vi "UpdateLowRateCount.vi"(7 "Qbus in":refnum<class "Qbus.lvclass">, 8 "error in (no error)":errorcluster, 10 "message value":variant, 11 "config":variant) -> (0 "error out":errorcluster, 3 "config out":variant)   [LabVIEW 2017, in "DataAccumulator.lvlib"]
uses:
  <vilib>/addons/InsightCM/Devices/Shared/Common/DataAccumulator/DataAccumulator.lvlib
  <vilib>/addons/Qbus/Qbus.lvclass
  <vilib>/addons/InsightCM/Devices/Shared/Common/DataAccumulator/controls/config.ctl
  <vilib>/addons/InsightCM/Devices/Shared/Common/DeviceHealth/controls/deviceHealthTag.ctl
  <vilib>/addons/InsightCM/Devices/Shared/Common/DeviceHealth/controls/SystemHealthTagEnum.ctl
  <vilib>/addons/InsightCM/MessageBus/Base/controls/Tag.ctl
  <vilib>/addons/InsightCM/MessageBus/Base/controls/KeyValuePair.ctl
  <vilib>/addons/InsightCM/MessageBus/Base/controls/TsTagValueString.ctl
  <vilib>/addons/InsightCM/MessageBus/Base/controls/TagValueUpdate.ctl
  <vilib>/addons/InsightCM/MessageBus/MessageLibrary/Tag/controls/TagUpdateTagValuesRoutedMessageBody.ctl
  <vilib>/addons/InsightCM/Devices/Shared/Common/ServerComm/ServerComm.lvlib
  <vilib>/addons/InsightCM/Devices/Shared/Common/DeviceHealth/DeviceHealth.lvlib
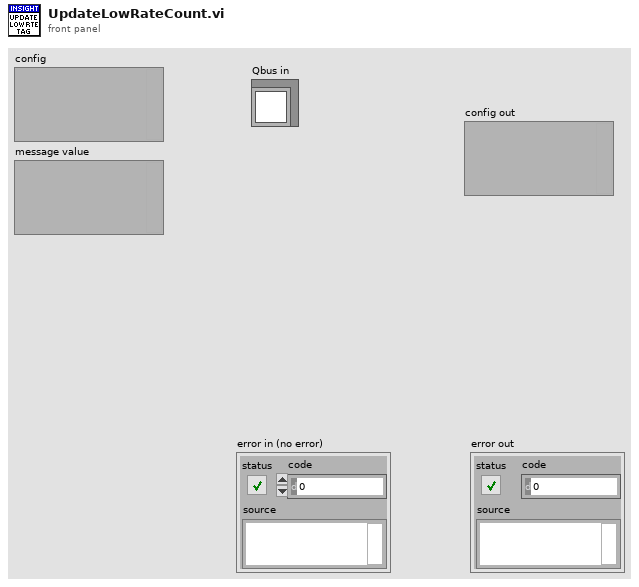
[diagram p1: front panel]
types:
  T1 = typedef "DataAccumulator.lvlib/config.ctl" = cluster{"Group":string, "BlockComplete":bool, "Ok To Start":bool, "Speed Ref Chan":string, "Current OpState":string, "MaxLowRateCPU(%)":dbl, "MaxLowRateMem(%)":dbl, "LowRateCount":i32, "LowRateCountTag":T2}
  T2 = typedef "DeviceHealth.lvlib/deviceHealthTag.ctl" = cluster{"SystemTags":T3, "TagId":string, "Tag":T4}
  T3 = typedef "DeviceHealth.lvlib/SystemHealthTagEnum.ctl" = enum16{"CPU Utilization", "Memory Utilization", "Disk Utilization", "Total Physical Memory", "Primary Disk Free", "Chassis Temperature", "LowRateCount"}
  T4 = typedef "Tag.ctl" = cluster{"Id":string, "Path":string, "Name":string, "Datatype":string, "Props":T5[], "Keywords":string[]}
  T5 = typedef "KeyValuePair.ctl" = cluster{"Key":string, "Value":string}
  T6 = typedef "TagValueUpdate.ctl" = cluster{"Tag":T4, "TsValue":T7}
  T7 = typedef "TsTagValueString.ctl" = cluster{"Value":string, "Timestamp":i64}
  T8 = typedef "TagUpdateTagValuesRoutedMessageBody.ctl" = cluster{"TagsValue":T6[]}
  T9 = typedef "Message.ctl" = cluster{"Header":T10, "Body":u8[]}
  T10 = typedef "MessageHeader.ctl" = cluster{"MessageName":string, "Timestamp":i64, "CorrelationId":string, "ContentType":string, "RoutingKey":string, "Properties":T5[]}
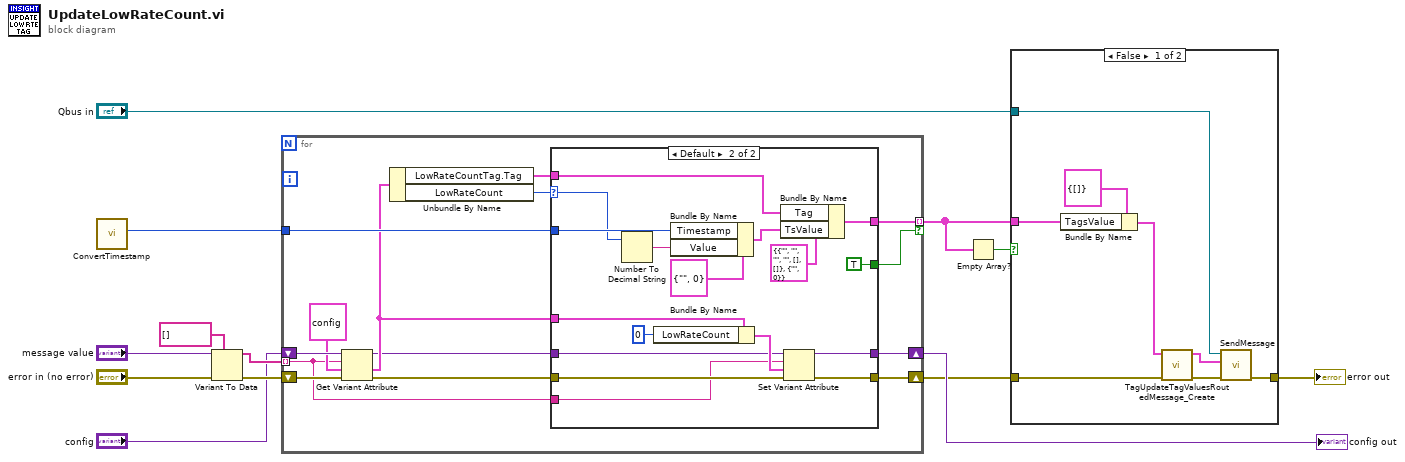
[diagram p0: block diagram]
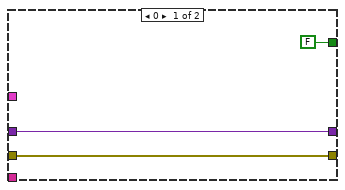
[diagram p2: hidden frame]
diagram:
  n1 = call <vilib>:"ConvertTimestamp.vi"() -> ("Timestamp out"=w3:i64)  [unwired: 11 in]
  n2 = Variant To Data(error in="error in (no error)", type=string[] [], Variant="message value") -> (data=w8:string[], error out=w10:errorcluster)
  n3 = for {
    shift-right: [w19] -> w2
    shift-left: w10 -> [w27]
    tunnel: w8 -> [w17] mode=indexing
    shift-right: [w18] -> w4
    shift-left: "config" -> [w26]
    tunnel: w3 -> [w24]
    tunnel: [w22] -> w1 mode=indexing if=w20
    n4 = Get Variant Attribute(Variant=w26, name=w17, default value (empty Variant)=T1 {"Group"="", "BlockComplete"=FALSE, "Ok To Start"=FALSE, "Speed Ref Chan"="", "Current OpState"="", "MaxLowRateCPU(%)"=0.0, "MaxLowRateMem(%)"=0.0, "LowRateCount"=0, "LowRateCountTag"={"SystemTags"=enum."CPU Utilization", "TagId"="", "Tag"={"Id"="", "Path"="", "Name"="", "Datatype"="", "Props"=[], "Keywords"=[]}}} ("Config"), error in=w27) -> (duplicate Variant=w15:variant, value=w16:T1, error out=w14:errorcluster)  [unwired: 1 out]
    n5 = Unbundle By Name(w16) -> ("LowRateCountTag.Tag"=w23:T4, "LowRateCount"=w21:i32)
    n6 = case shown="Default" w21 {
      selector: w21 -> [_ w39]
      tunnel: w24 -> [_ w44]
      tunnel: w23 -> [_ w42]
      tunnel: [_ w41] -> w22
      tunnel: [FALSE TRUE] -> w20
      tunnel: w14 -> [w28 w36]
      tunnel: [w28 w35] -> w19
      tunnel: w15 -> [w29 w34]
      tunnel: [w29 w33] -> w18
      tunnel: w17 -> [_ w32]
      tunnel: w16 -> [_ w31]
      frame 0 {
      }
      frame Default {
        n7 = Number To Decimal String(number=w39) -> (decimal integer string=w43:string)  [unwired: 1 in]
        n8 = Bundle By Name(cluster=w31, "LowRateCount"=0) -> (w38:T1)
        n9 = Bundle By Name(cluster=T7 {"Value"="", "Timestamp"=0} ("TsValue"), "Timestamp"=w44, "Value"=w43) -> (w45:T7)
        n10 = Bundle By Name(cluster=T6 {"Tag"={"Id"="", "Path"="", "Name"="", "Datatype"="", "Props"=[], "Keywords"=[]}, "TsValue"={"Value"="", "Timestamp"=0}} ("TagValue"), "Tag"=w42, "TsValue"=w45) -> (w41:T6)
        n11 = Set Variant Attribute(Variant=w34, name=w32, value=w38, error in=w36) -> (Variant out=w33:variant, error out=w35:errorcluster)  [unwired: 1 out]
      }
    }
  }
  "config out" <- w4
  n12 = Empty Array?(array=w1) -> (empty?=w13:bool)
  n13 = case shown="False" w13 {
    tunnel: w2 -> [w51 w56]
    tunnel: [w55 w56] -> w11
    tunnel: w1 -> [w52 _]
    tunnel: "Qbus in" -> [w54 _]
    frame False {
      n14 = Bundle By Name(cluster=T8 {"TagsValue"=[]} ("TagUpdateTagValuesRoutedMessage"), "TagsValue"=w52) -> (w49:T8)
      n15 = call <vilib>:"TagUpdateTagValuesRoutedMessage_Create.vi"("error in (no error)"=w51, "TagUpdateTagValuesRoutedMessage"=w49) -> ("error out"=w50:errorcluster, "Message"=w48:T9)  [unwired: 8 in]
      n16 = call <vilib>:"SendMessage.vi"("error in (no error)"=w50, "message"=w48, "Qbus in"=w54) -> ("error out"=w55:errorcluster)  [unwired: 7 in, 1 out]
    }
    frame True {
    }
  }
  "error out" <- w11
